vi "Wfm_skaluj_osX.vi"(7 "size(s)":dbl, 8 "error in (no error)":errorcluster, 10 "Zakres wysw":dbl, 11 "Waveform in":refnum<vi>) -> (0 "error out":errorcluster)   [LabVIEW 2013]
doc: "Skaluje oś X przebiegów na Waveform Graph\nWartość 0 wyłącza skalowanie - cały zakres od wartości 0"
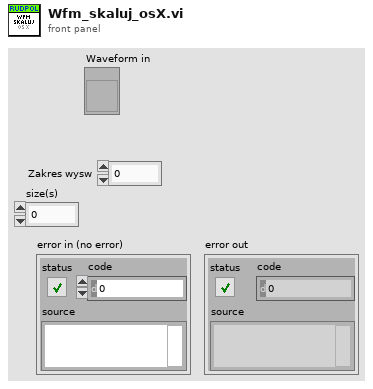
[diagram p1: front panel]
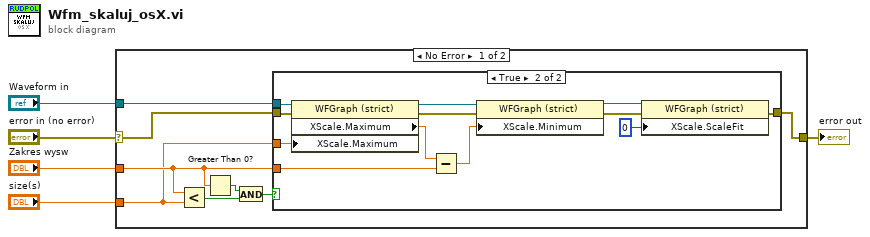
[diagram p0: block diagram]
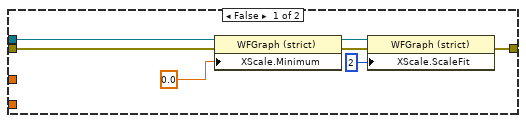
[diagram p2: hidden frame]
diagram:
  n1 = case shown="No Error" "error in (no error)" {
    selector: "error in (no error)" -> [w11 w33]
    tunnel: "Zakres wysw" -> [w7 _]
    tunnel: "Waveform in" -> [w12 _]
    tunnel: [w13 w33] -> w3
    tunnel: "size(s)" -> [w6 _]
    frame No Error {
      n2 = Less?(x=w7, y=w6) -> (x < y?=w10:bool)
      n3 = Greater Than 0?(x=w7) -> (x > 0?=w8:bool)
      n4 = And(x=w8, y=w10) -> (x .and. y?=w9:bool)
      n5 = case shown="True" w9 {
        tunnel: w11 -> [w15 w31]
        tunnel: w12 -> [w16 w30]
        tunnel: [w17 w23] -> w13
        tunnel: w7 -> [_ w32]
        tunnel: w6 -> [_ w22]
        frame False {
          n6 = property on="Property Node" class="WFGraph (strict)"(reference=w16, error in=w15, "XScale.Minimum"=0.0 ("X Scale.Range:Minimum")) -> (reference out=w19:refnum<vi>, error out=w18:errorcluster)
          n7 = property on="Property Node" class="WFGraph (strict)"(reference=w19, error in=w18, "XScale.ScaleFit"=u8 2 ("X Scale.Scale Fit")) -> (error out=w17:errorcluster)  [unwired: 1 out]
        }
        frame True {
          n8 = property on="Property Node" class="WFGraph (strict)"(reference=w30, error in=w31, "XScale.Maximum"=w22) -> (reference out=w27:refnum<vi>, error out=w28:errorcluster, "XScale.Maximum"=w21:dbl)
          n9 = Subtract(x=w21, y=w32) -> (x-y=w29:dbl)
          n10 = property on="Property Node" class="WFGraph (strict)"(reference=w27, error in=w28, "XScale.Minimum"=w29) -> (reference out=w24:refnum<vi>, error out=w25:errorcluster)
          n11 = property on="Property Node" class="WFGraph (strict)"(reference=w24, error in=w25, "XScale.ScaleFit"=u8 0 ("X Scale.Scale Fit")) -> (error out=w23:errorcluster)  [unwired: 1 out]
        }
      }
    }
    frame Error {
    }
  }
  "error out" <- w3
